vi "Close.vi"(8 "error in (no error)":errorcluster, 11 "Mettler Settings in":T1) -> (0 "error out":errorcluster, 3 "Mettler Settings out":T1)   [LabVIEW 2018, in "Mettler Toledo.lvlib"]
uses:
  Mettler Toledo.lvlib
  Controls/Settings Cluster.ctl
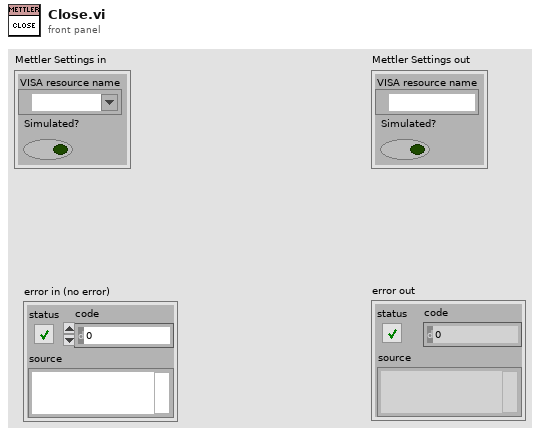
[diagram p1: front panel]
types:
  T1 = typedef "Mettler Toledo.lvlib/Settings Cluster.ctl" = cluster{"VISA resource name":refnum<visa-resource-name>, "Simulated?":bool}
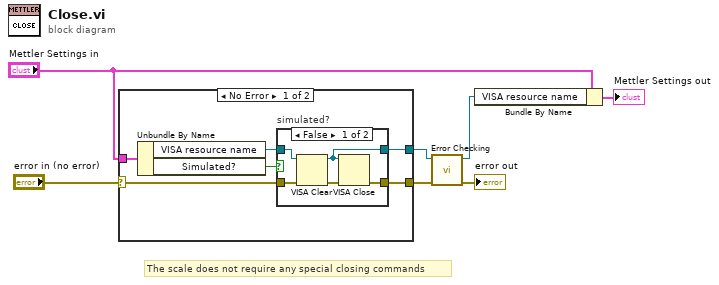
[diagram p0: block diagram]
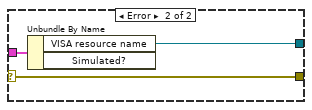
[diagram p3: hidden frame]
diagram:
  # "The scale does not require any special closing commands"
  n1 = case shown="No Error" "error in (no error)" {
    selector: "error in (no error)" -> [w12 w23]
    tunnel: [w11 w23] -> w2
    tunnel: "Mettler Settings in" -> [w10 w22]
    tunnel: [w8 w21] -> w4
    frame No Error {
      n2 = Unbundle By Name(w10) -> ("VISA resource name"=w9:refnum<visa-resource-name>, "Simulated?"=w13:bool)
      n3 = case "simulated?" shown="False" w13 {
        tunnel: [w18 w20] -> w11
        tunnel: w12 -> [w16 w20]
        tunnel: [w14 w19] -> w8
        tunnel: w9 -> [w17 w19]
        frame False {
          n4 = VISA Clear(VISA resource name=w17, error in (no error)=w16) -> (VISA resource name out=w14:refnum<visa-resource-name>, error out=w15:errorcluster)
          n5 = VISA Close(VISA resource name=w14, error in (no error)=w15) -> (error out=w18:errorcluster)
        }
        frame True {
        }
      }
    }
    frame Error {
      n6 = Unbundle By Name(w22) -> ("VISA resource name"=w21:refnum<visa-resource-name>)  [unwired: 1 out]
    }
  }
  n7 = call "Error Checking.vi"("error in (no error)"=w2, "VISA resource name"=w4) -> ("error out"=→"error out":errorcluster, "VISA resource name"=w3:refnum<visa-resource-name>)  [unwired: 7 in, 1 out]
  n8 = Bundle By Name(cluster="Mettler Settings in", "VISA resource name"=w3) -> (→"Mettler Settings out":T1)
